vi "mlink_dsp_init.vi"(7 "DSP binary path":path, 8 "error in (no error)":errorcluster, 9 "rate [period s]":dbl=0.1, 10 "duration [s]":dbl=0.1, 11 "connection ID":i32=-1) -> (0 "error out":errorcluster, 3 "connection ID out":i32)   [LabVIEW 2009, in "MicroDAQ.lvlib" / "mlink.lvlib"]
doc: "This function loads program generated for MicroDAQ DSP processor. The function can be used with DSP executables generated from Xcos model only. It loads binary file from path pointed by dsp_binary_path. The function can modify Xcos model steps per seconds rate by setting rate argument. This way user can run generated DSP program with different model step rate without a need to re-generated DSP executable. If rate is equal -1 Xcos model step rate setting will be not overwritten. The duration parameter modifies Xcos model lifetime, value of -1 means model will run infinitely."
uses:
  <instrlib>/MicroDAQ/Mlink library wraper/mlink.lvlib
  <instrlib>/MicroDAQ/MLink32.dll
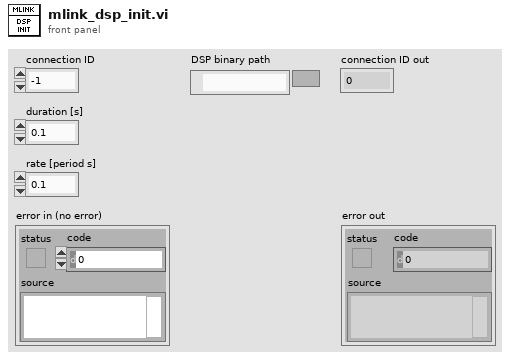
[diagram p1: front panel]
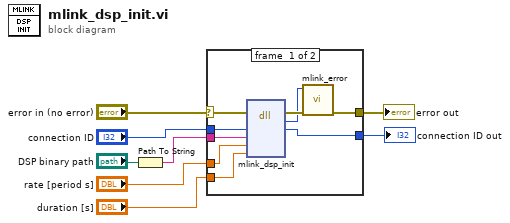
[diagram p0: block diagram]
diagram:
  n1 = Path To String(path="DSP binary path") -> (string=w7:string)
  n2 = case shown="No Error" "error in (no error)" {
    selector: "error in (no error)" -> [w17 w19]
    tunnel: w7 -> [w16 _]
    tunnel: "connection ID" -> [w15 w18]
    tunnel: "duration [s]" -> [w14 _]
    tunnel: [w13 w18] -> w4
    tunnel: [w10 w19] -> w2
    tunnel: "rate [period s]" -> [w9 _]
    frame #0 {
      n3 = dll-call lib="C:/Program Files (x86)/National Instruments/LabVIEW 2009/instr.lib/MicroDAQ/MLink32.dll" fn="mlink_dsp_init" ("MLink64.dll:mlink_dsp_run")(error in=w17, "link_fd"=w15, "dsp_binary_path"=w16, "rate"=w9, "duration"=w14) -> (error out=w12:errorcluster, "return type"=w11:i32, "link_fd"=w13:i32)  [unwired: 5 in, 1 out]
      n4 = call <instrlib>:"mlink_error.vi"("error in (no error)"=w12, "error code"=w11) -> ("error out"=w10:errorcluster)  [unwired: 9 in]
    }
    frame #1 {
    }
  }
  "connection ID out" <- w4
  "error out" <- w2
